vi "Launcher.vi"(8 "error in (no error)":errorcluster, 10 "Log Class":refnum<class "Build_Javier_Lopez_lib_Configuration_Filejson class.lvclass">, 11 "Module Communication in":refnum<class "Communication.lvclass">) -> (0 "error out":errorcluster)   [LabVIEW 2021, in "Communication.lvclass"]
uses:
  Communication.lvclass
  <vilib>/Javier Lopez/Configuration File/Json Element/Build_Javier_Lopez_lib_Configuration_Filejson class.lvclass
  Module Launcher Base/Launcher Base.lvclass
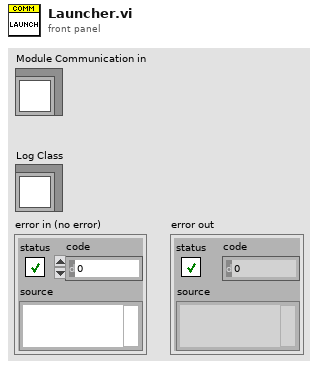
[diagram p1: front panel]
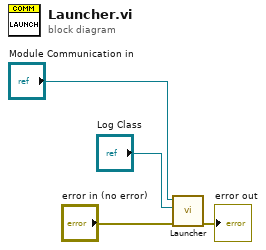
[diagram p0: block diagram]
diagram:
  n1 = call-parent "Launcher.vi"("error in (no error)"="error in (no error)", "Log Class"="Log Class", "Module Launcher Base in"="Module Communication in") -> ("error out"=→"error out":errorcluster)  [unwired: 8 in]
